vi "GetPositionUm.vi"(8 "error in (no error)":errorcluster, 10 "Stage Label":string, 11 "DemoStage in":refnum<class "DemoStage.lvclass">) -> (0 "error out":errorcluster, 2 "Stage Position":dbl, 3 "DemoStage out":refnum<class "DemoStage.lvclass">)   [LabVIEW 2020, in "DemoStage.lvlib" / "DemoStage.lvclass"]
uses:
  DemoStage.lvclass
  DemoStage.lvclass/DemoStage.ctl
  <vilib>/numeric/Random Number (Range) DBL.vi
  Hardware Abstraction Layer/Component/Stage/Stage/Stage.lvclass
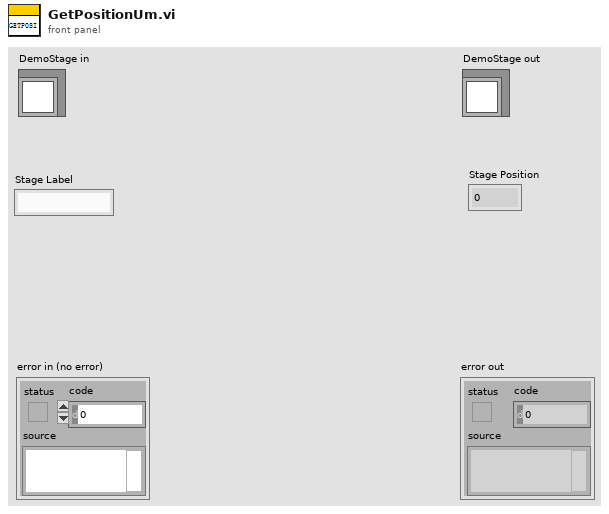
[diagram p1: front panel]
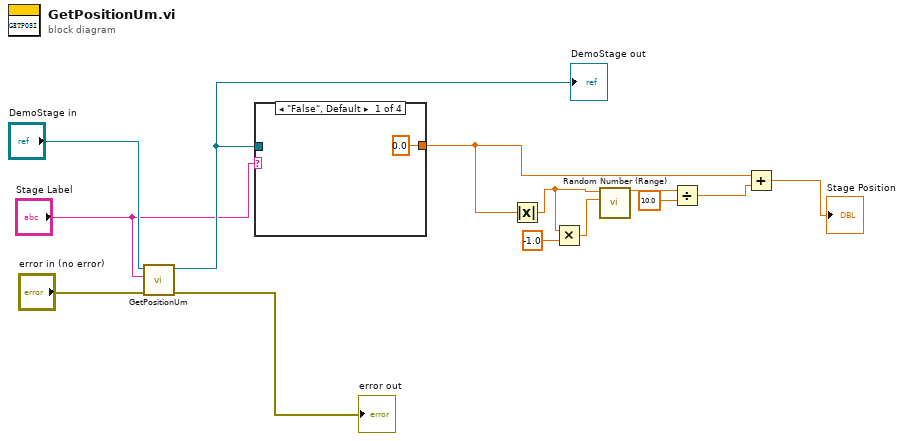
[diagram p0: block diagram]
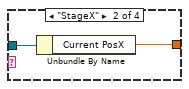
[diagram p2: hidden frame]
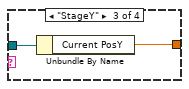
[diagram p3: hidden frame]
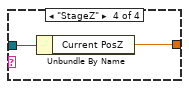
[diagram p4: hidden frame]
diagram:
  n1 = call-parent "GetPositionUm.vi"("error in (no error)"="error in (no error)", "Stage Label"="Stage Label", "Stage in"="DemoStage in") -> ("error out"=→"error out":errorcluster, "Stage out"=w10:refnum<class "DemoStage.lvclass">)  [unwired: 6 in, 1 out]
  "DemoStage out" <- w10
  n2 = case shown="\"False\", Default" "Stage Label" {
    tunnel: w10 -> [_ w16 w18 w20]
    tunnel: [0.0 ("Current PosZ") w15 w17 w19] -> w4
    frame "False", Default {
    }
    frame "StageX" {
      n3 = Unbundle By Name(w16) -> ("Current PosX"=w15:dbl)
    }
    frame "StageY" {
      n4 = Unbundle By Name(w18) -> ("Current PosY"=w17:dbl)
    }
    frame "StageZ" {
      n5 = Unbundle By Name(w20) -> ("Current PosZ"=w19:dbl)
    }
  }
  n6 = Absolute Value(x=w4) -> (abs(x)=w7:dbl)
  n7 = Multiply(x=w7, y=-1.0) -> (x*y=w8:dbl)
  n8 = call-poly <vilib>:"Random Number (Range).vi"("lower bound (0)"=w8, "upper bound (100)"=w7) -> ("number"=w6:dbl)  [unwired: 9 in]
  n9 = Divide(x=w6, y=10.0) -> (x/y=w3:dbl)
  n10 = Add(x=w4, y=w3) -> (x+y=→"Stage Position":dbl)
